vi "Graph.vi"(6 "Ring size (points) (1024)":u32=1024, 8 "error in (no error)":errorcluster, 9 "Store Ring? (f)":bool, 10 "Store History? (f)":bool, 11 "Readable in":refnum<class "Readable.lvclass">) -> (0 "error out":errorcluster, 1 "Ring Buffers":T5, 2 "History Buffers":T5, 3 "Readable out":refnum<class "Readable.lvclass">, 5 "Data Points":T1)   [LabVIEW 2009, in "Readable.lvclass"]
doc: "(Dynamic) Take a data point, then append it to an internal history buffer. Return the history buffer as a waveform array configured for graphing."
uses:
  Readable.lvclass
  TX Graph.ctl
  Data Points.ctl
  Data Point.ctl
  Time.ctl
  X.ctl
  Readable.lvclass/Readable.ctl
panel:
  # "Generate a waveform array for graphing."
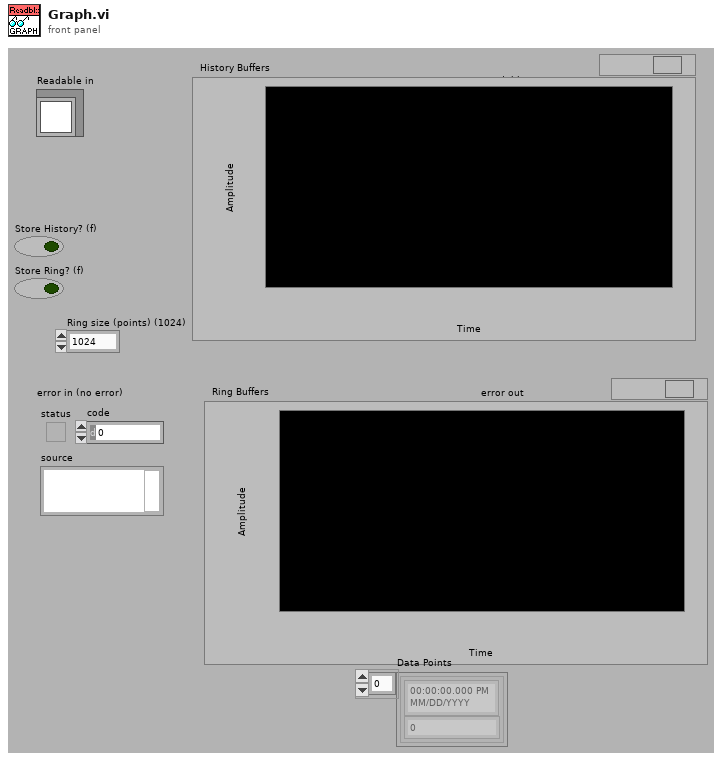
[diagram p1: front panel]
types:
  T1 = typedef "Readable.lvclass/Data Points.ctl" = T2[]
  T2 = typedef "Readable.lvclass/Data Point.ctl" = cluster{"t":T3, "x":T4}
  T3 = typedef "Readable.lvclass/Time.ctl" = timestamp
  T4 = typedef "Readable.lvclass/X.ctl" = dbl
  T5 = typedef "Readable.lvclass/TX Graph.ctl" = cluster{"Data Points":cluster{"t":timestamp, "x":dbl}[]}[]
  T6 = typedef "Readable.lvclass/Data Channels.ctl" = T7[]
  T7 = typedef "Readable.lvclass/Data Channel.ctl" = cluster{"Name":string, "Data Point":T2, "Unit":string}
  T8 = typedef "Readable.lvclass/Channel Names.ctl" = string[]
  T9 = cluster{"Data Points":cluster{"t":timestamp, "x":dbl}[]}
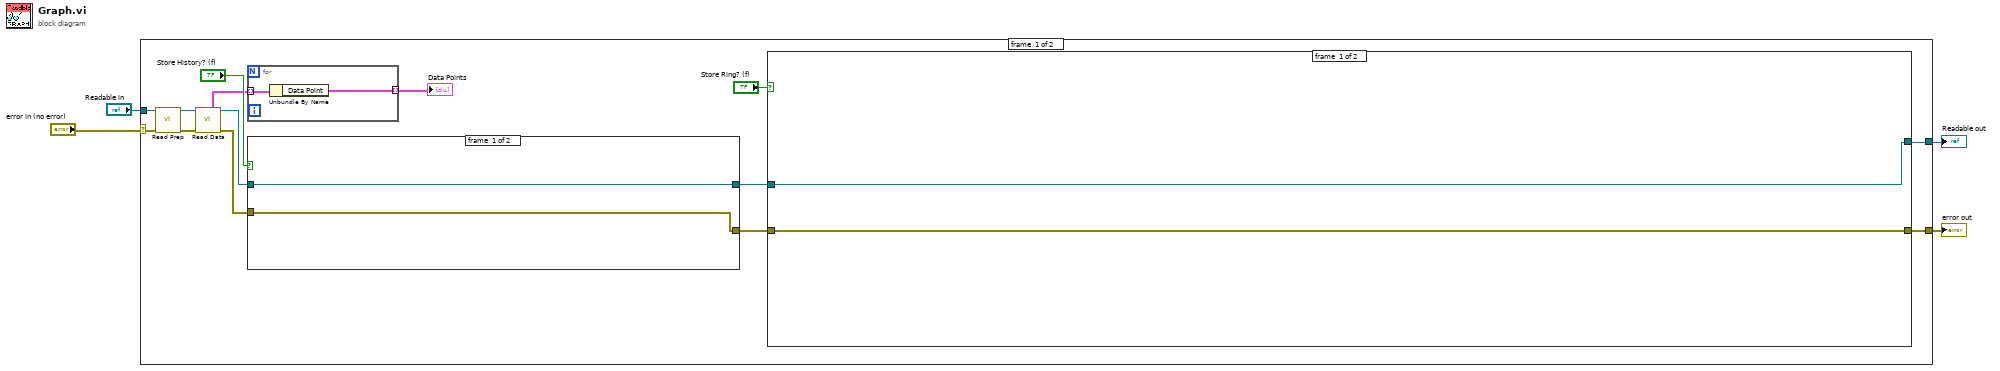
[diagram p0: block diagram]
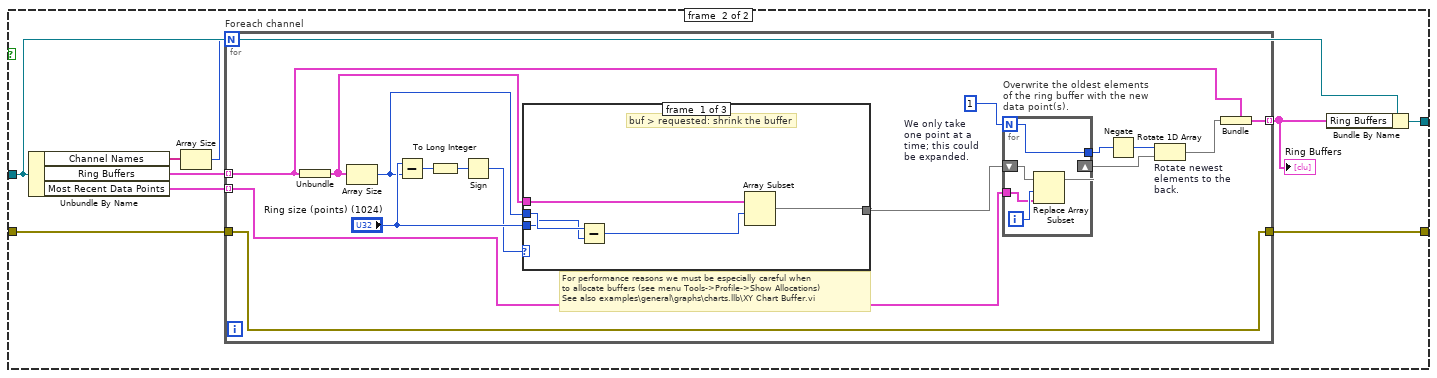
[diagram p2: hidden frame]
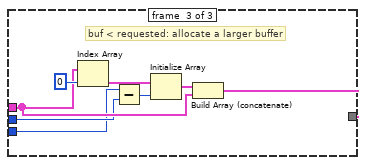
[diagram p4: hidden frame]
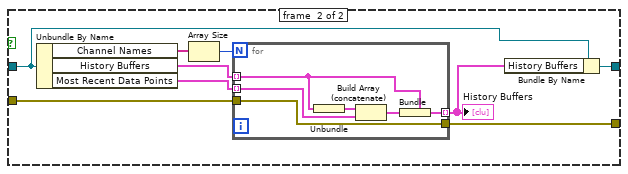
[diagram p5: hidden frame]
diagram:
  n1 = case shown="No Error" "error in (no error)" {
    selector: "error in (no error)" -> [w8 w85]
    tunnel: [w13 w85] -> w3
    tunnel: [w15 w84] -> w1
    tunnel: "Readable in" -> [w5 w84]
    frame #0 {
      n2 = call-dynamic "Read Prep.vi"("error in (no error)"=w8, "Readable in"=w5) -> ("error out"=w7:errorcluster, "Readable out"=w6:refnum<class "Readable.lvclass">)  [unwired: 8 in]
      n3 = call "Read Data.vi"("error in (no error)"=w7, "Readable in"=w6) -> ("error out"=w11:errorcluster, "Readable out"=w12:refnum<class "Readable.lvclass">, "Data Channels"=w10:T6)  [unwired: 3 in, 4 out]
      n4 = for {
        tunnel: w10 -> [w20] mode=indexing
        tunnel: [w19] -> w9 mode=indexing
        n5 = Unbundle By Name(w20) -> ("Data Point"=w19:T2)
      }
      "Data Points" <- w9
      n6 = case shown="True" "Store History? (f)" {
        tunnel: [w68 w77] -> w16
        tunnel: [w67 w76] -> w14
        tunnel: w11 -> [w67 w73]
        tunnel: w12 -> [w68 w71]
        frame #0 {
        }
        frame #1 {
          n7 = Unbundle By Name(w71) -> ("Channel Names"=w70:T8, "History Buffers"=w75:T5, "Most Recent Data Points"=w72:T1)
          n8 = Array Size(array=w70) -> (size(s)=w69:i32)
          n9 = for {
            N: w69 -> [_]
            tunnel: w73 -> [w83]
            tunnel: [w83] -> w76
            tunnel: [w81] -> w74 mode=indexing
            tunnel: w75 -> [w80] mode=indexing
            tunnel: w72 -> [w78] mode=indexing
            n10 = Unbundle(w80) -> ("Data Points"=w79:cluster{"t":timestamp, "x":dbl}[])
            n11 = Build Array (concatenate)(w79, w78) -> (w82:T2[])
            n12 = Bundle(cluster=w80, "Data Points"=w82) -> (w81:T9)
          }
          "History Buffers" <- w74
          n13 = Bundle By Name(cluster=w71, "History Buffers"=w74) -> (w77:refnum<class "Readable.lvclass">)
        }
      }
      n14 = case shown="True" "Store Ring? (f)" {
        tunnel: [w22 w31] -> w15
        tunnel: [w21 w30] -> w13
        tunnel: w14 -> [w21 w28]
        tunnel: w16 -> [w22 w26]
        frame #0 {
        }
        frame #1 {
          n15 = Unbundle By Name(w26) -> ("Channel Names"=w23:T8, "Ring Buffers"=w24:T5, "Most Recent Data Points"=w27:T1)
          n16 = Array Size(array=w23) -> (size(s)=w25:i32)
          n17 = for "Foreach channel" {
            N: w25 -> [_]
            tunnel: w28 -> [w47]
            tunnel: [w47] -> w30
            tunnel: [w46] -> w29 mode=indexing
            tunnel: w24 -> [w45] mode=indexing
            tunnel: w27 -> [w38] mode=indexing
            w37 = 1  # We only take one point at a time; this could be expanded.
            # "For performance reasons we must be especially careful when\nto allocate buffers (see menu Tools->Profile->Show Allocations)\nSee also examples\\general\\graphs\\charts.llb\\XY Chart Buffer.vi"
            n18 = Unbundle(w45) -> ("Data Points"=w44:cluster{"t":timestamp, "x":dbl}[])
            n19 = Array Size(array=w44) -> (size(s)=w41:i32)
            n20 = Subtract(x="Ring size (points) (1024)", y=w41) -> (x-y=w43:u32)
            n21 = To Long Integer(number=w43) -> (32bit integer=w40:i32)
            n22 = Sign(1:w40) -> (0:w39:i32)
            n23 = case shown="1.." w39 {
              tunnel: [w56 w58 w62] -> w33
              tunnel: w44 -> [w57 w58 w63]
              tunnel: "Ring size (points) (1024)" -> [w54 _ w60]
              tunnel: w41 -> [w55 _ w61]
              frame #0 {
                # "buf > requested: shrink the buffer"
                n24 = Subtract(x=w55, y=w54) -> (x-y=w53:u32)
                n25 = Array Subset(array=w57, index=w53) -> (w56:cluster{"t":timestamp, "x":dbl}[])  [unwired: 1 in]
              }
              frame #1 {
                # "buf == requested"
              }
              frame #2 {
                # "buf < requested: allocate a larger buffer"
                n26 = Index Array(array=w63, index=0) -> (element=w65:cluster{"t":timestamp, "x":dbl})
                n27 = Subtract(x=w60, y=w61) -> (x-y=w59:u32)
                n28 = Initialize Array(w65, w59) -> (w64:cluster{"t":timestamp, "x":dbl}[])
                n29 = Build Array (concatenate)(w64, w63) -> (w62:cluster{"t":timestamp, "x":dbl}[])
              }
            }
            n30 = for "Overwrite the oldest elements\nof the ring buffer with the new\ndata point(s)." {
              N: w37 -> [w52]
              shift-right: [w48] -> w34
              shift-left: w33 -> [w49]
              tunnel: w38 -> [w50]
              tunnel: [w52] -> w36
              i -> [w51]
              n31 = Replace Array Subset(array=w49, new element=w50, index=w51) -> (w48:cluster{"t":timestamp, "x":dbl}[])
            }
            n32 = Negate(x=w36) -> (-x=w35:i32)
            n33 = Rotate 1D Array "Rotate newest \nelements to the \nback."(1:w34, 2:w35) -> (0:w32:cluster{"t":timestamp, "x":dbl}[])
            n34 = Bundle(cluster=w45, "Data Points"=w32) -> (w46:T9)
          }
          "Ring Buffers" <- w29
          n35 = Bundle By Name(cluster=w26, "Ring Buffers"=w29) -> (w31:refnum<class "Readable.lvclass">)
        }
      }
    }
    frame #1 {
    }
  }
  "error out" <- w3
  "Readable out" <- w1
